vi "run.vi"(8 "error in (no error)":errorcluster, 10 "Path":path, 11 "settingsViewer in":refnum<class "settingsViewer.lvclass">) -> (0 "error out":errorcluster, 3 "settingsViewer out":refnum<class "settingsViewer.lvclass">)   [LabVIEW 2009, in "Views.lvlib" / "SettingsViewer.lvclass"]
uses:
  settingsViewer.lvclass
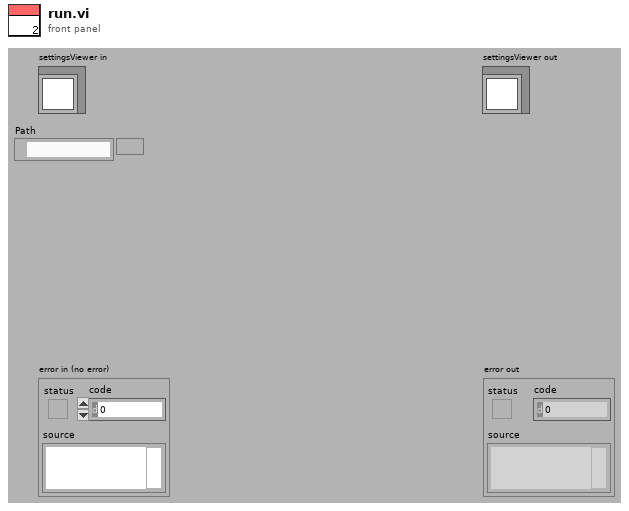
[diagram p1: front panel]
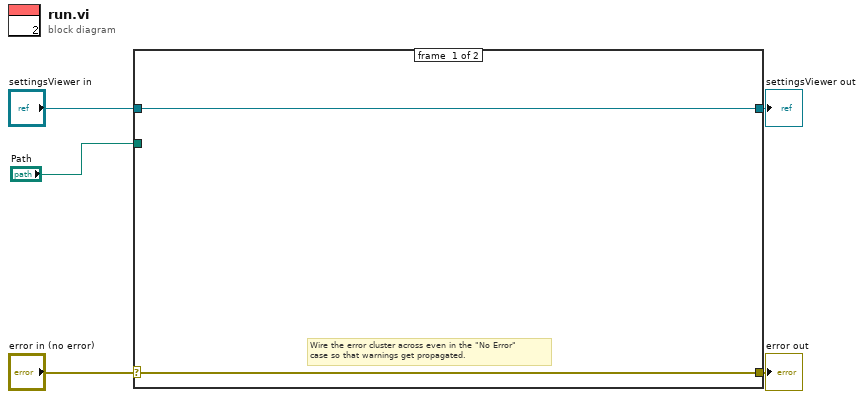
[diagram p0: block diagram]
diagram:
  n1 = case shown="No Error" "error in (no error)" {
    selector: "error in (no error)" -> [w6 w9]
    tunnel: [w6 w9] -> w4
    tunnel: [w7 w8] -> w2
    tunnel: "settingsViewer in" -> [w7 w8]
    tunnel: "Path" -> [_ _]
    frame #0 {
      # "Wire the error cluster across even in the \"No Error\"\ncase so that warnings get propagated."
    }
    frame #1 {
    }
  }
  "error out" <- w4
  "settingsViewer out" <- w2
